vi "LV_client_port_DAQ - sh 4 outputs.vi"() -> ()   [LabVIEW 2014]
uses:
  <vilib>/DAQmx/create/channels.llb/DAQmx Create Channel (AO-Voltage-Basic).vi
  <vilib>/DAQmx/configure/timing.llb/DAQmx Timing (Sample Clock).vi
  <vilib>/DAQmx/configure/trigger.llb/DAQmx Start Trigger (None).vi
  <vilib>/DAQmx/write.llb/DAQmx Write (Analog 1D DBL NChan 1Samp).vi
panel:
  in  "mode":T1(ring)=enum."Immediate"
  in  "Yaw Constant":dbl=1800.0
  in  "Forward Constnt":dbl=1800.0
  out "Forward":dbl(graph)
  out "Yaw":dbl(graph)
  in  "Vthresh":dbl=0.1
  in  "forward\noffset":dbl=-0.019 format="%_4f"
  in  "Yaw\nOffset":dbl=-0.019 format="%_4f"
  out "Forward 2":dbl(graph)
  out "Yaw 2":dbl(graph)
  in  "Stop":bool
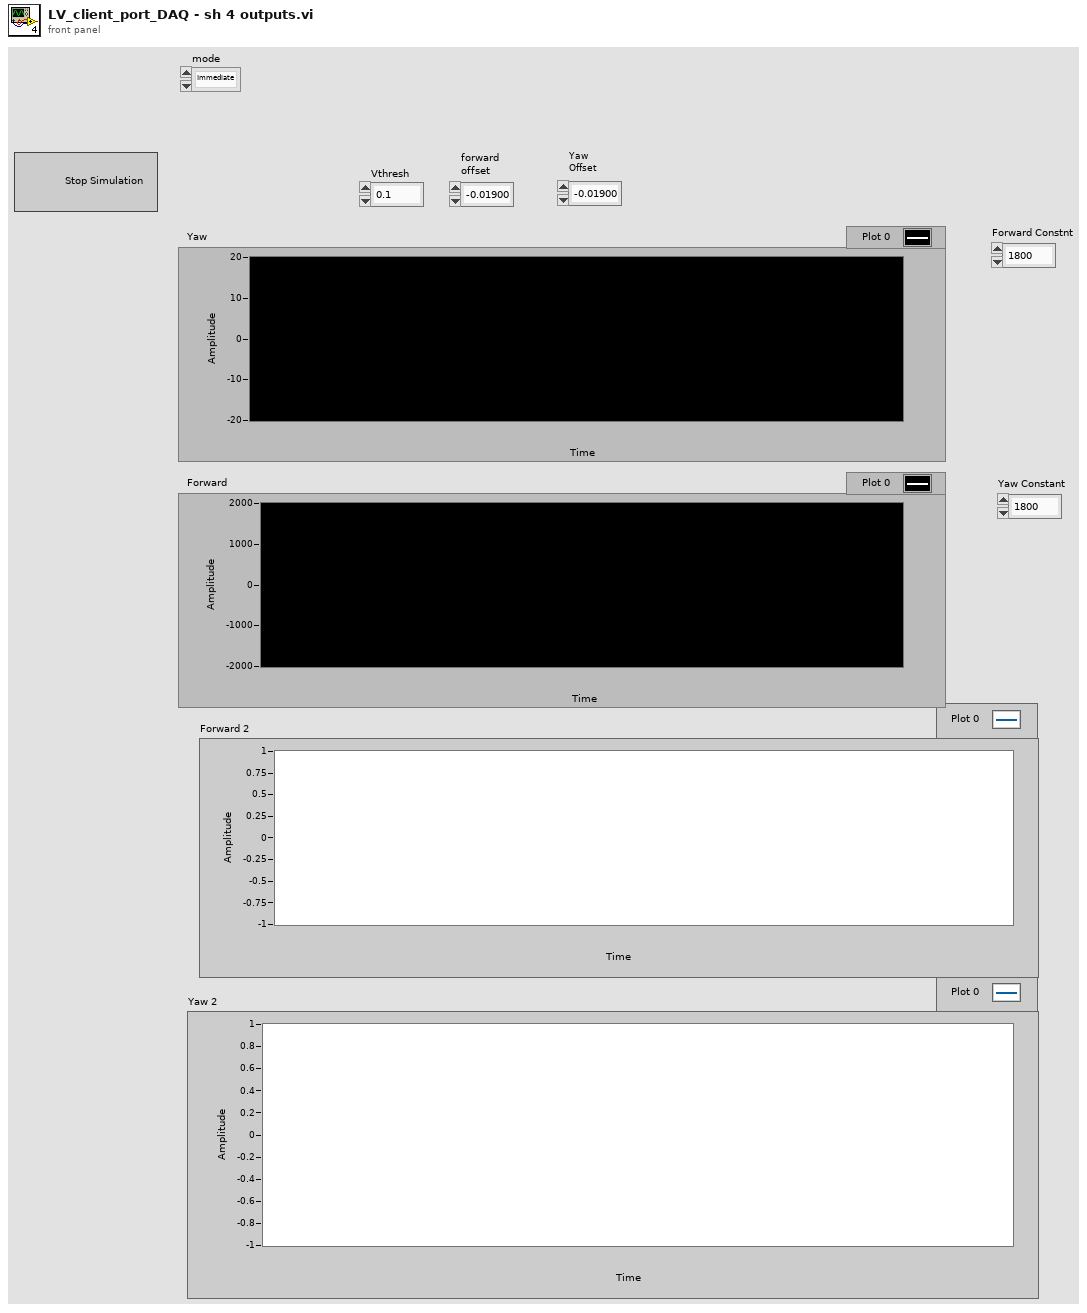
[diagram p1: front panel]
types:
  T1 = enum16{"Standard", "Buffered", "CRLF", "Immediate"}
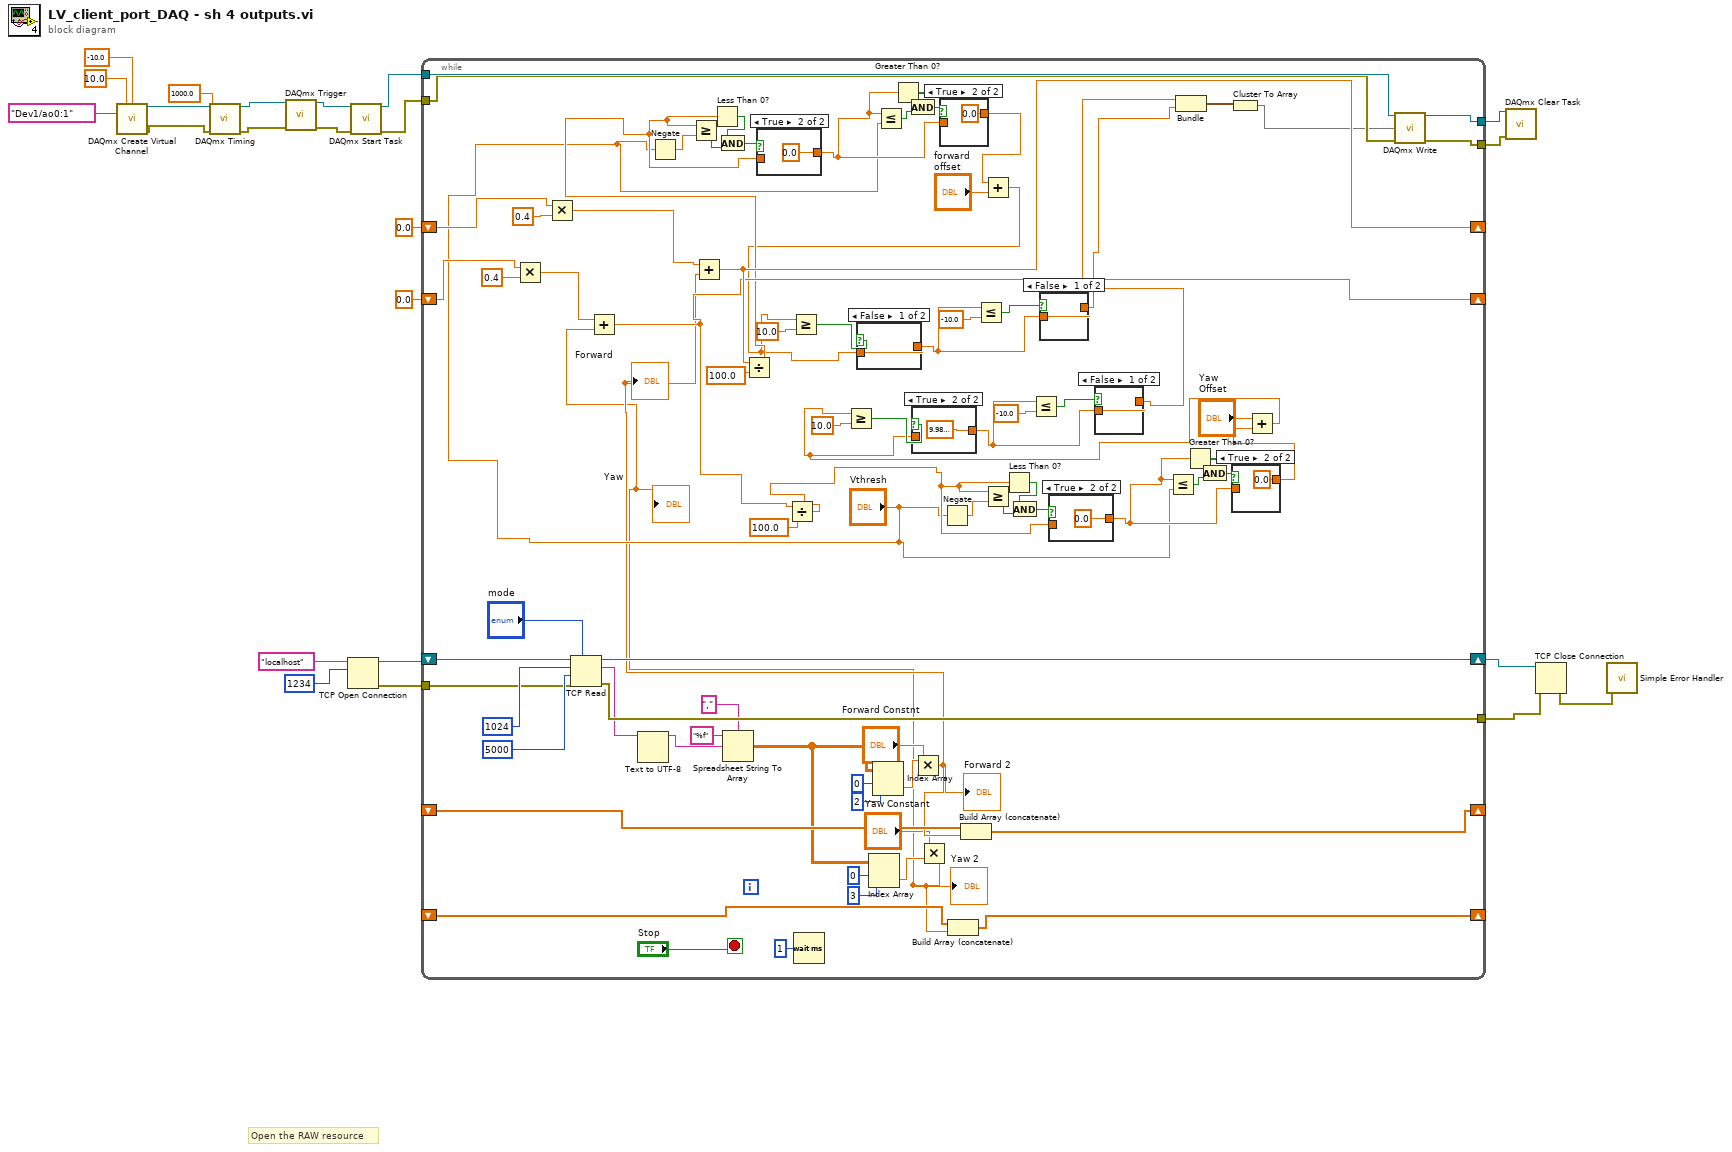
[diagram p0: block diagram]
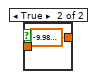
[diagram p6: hidden frame]
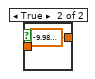
[diagram p8: hidden frame]
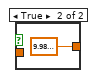
[diagram p9: hidden frame]
diagram:
  # "Open the RAW resource"
  n1 = call-poly <vilib>:"DAQmx Create Virtual Channel.vi"("maximum value"=10.0, "minimum value"=-10.0, "physical channels"=tag "Dev1/ao0:1") -> ("task out"=w21:refnum<k21>, "error out"=w20:errorcluster)  [unwired: 11 in]
  n2 = call-poly <vilib>:"DAQmx Timing.vi"("task/channels in"=w21, "rate"=1000.0, "error in"=w20) -> ("task out"=w19:refnum<k21>, "error out"=w18:errorcluster)  [unwired: 11 in]
  n3 = call-poly <vilib>:"DAQmx Trigger.vi"("task/channels in"=w19, "error in"=w18) -> ("task out"=w17:refnum<k21>, "error out"=w16:errorcluster)  [unwired: 12 in]
  n4 = TCP Open Connection(address="localhost", remote port or service name=u16 1234) -> (connection ID=w5:refnum<k5>, error out=w4:errorcluster)  [unwired: 3 in]
  n5 = call <vilib>:"DAQmx Start Task.vi"("task/channels in"=w17, "error in"=w16) -> ("task out"=w11:refnum<k21>, "error out"=w10:errorcluster)  [unwired: 12 in]
  n6 = while {
    shift-right: [w90] -> _
    shift-left: 0.0 -> [w91]
    shift-right: [w86] -> _
    shift-left: 0.0 -> [w87]
    tunnel: w11 -> [w59]
    tunnel: w10 -> [w58]
    tunnel: [w61] -> w9
    tunnel: [w60] -> w8
    tunnel: [w41] -> w3
    shift-right: [w40] -> w1
    shift-left: w5 -> [w46]
    shift-right: [w50] -> _
    shift-left: _ -> [w51]
    shift-right: [w48] -> _
    shift-left: _ -> [w49]
    tunnel: w4 -> [w43]
    stop <- "Stop" stop-if-true
    n7 = Multiply(x=w87, y=0.4) -> (x*y=w89:dbl)
    n8 = Multiply(x=w91, y=0.4) -> (x*y=w93:dbl)
    n9 = TCP Read(connection ID=w46, bytes to read=1024, error in (no error)=w43, 7:"mode", 9:5000 ("timeout ms (25000)")) -> (connection ID out=w40:refnum<k5>, data out=w39:string, error out=w41:errorcluster)
    n10 = Text to UTF-8(11:w39) -> (3:w38:string)  [unwired: 2 in, 1 out]
    n11 = Negate(x="Vthresh") -> (-x=w77:dbl)
    n12 = Spreadsheet String To Array(delimiter (Tab)=",", format string="%f", spreadsheet string=w38) -> (array=w33:dbl[][])  [unwired: 1 in]
    n13 = Wait (ms)(milliseconds to wait=u32 1) -> ()  [unwired: 1 out]
    n14 = Index Array(array=w33, index (row)=0, index (col)=3 ("disabled index (col)")) -> (element=w27:dbl)
    n15 = Index Array(array=w33, index (row)=0, index (col)=2 ("disabled index (col)")) -> (element=w30:dbl)
    n16 = Multiply(x=w30, y="Forward Constnt") -> (x*y=w28:dbl)
    "Forward" <- w28
    "Forward 2" <- w28
    n17 = Add(x=w93, y=w28) -> (x+y=w90:dbl)
    n18 = Divide(x=w90, y=sgl 100.0) -> (x/y=w68:dbl)
    n19 = Greater Or Equal?(x=w68, y=w77) -> (x >= y?=w74:bool)
    n20 = Less Than 0?(x=w68) -> (x < 0?=w75:bool)
    n21 = And(x=w75, y=w74) -> (x .and. y?=w76:bool)
    n22 = case shown="True" w76 {
      tunnel: [w107 sgl 0.0 ("y")] -> w73
      tunnel: w68 -> [w107 _]
      frame False {
      }
      frame True {
      }
    }
    n23 = Less Or Equal?(x=w73, y="Vthresh") -> (x <= y?=w71:bool)
    n24 = Greater Than 0?(x=w73) -> (x > 0?=w72:bool)
    n25 = And(x=w72, y=w71) -> (x .and. y?=w70:bool)
    n26 = Multiply(x="Yaw Constant", y=w27) -> (x*y=w25:dbl)
    "Yaw" <- w25
    "Yaw 2" <- w25
    n27 = Add(x=w89, y=w25) -> (x+y=w86:dbl)
    n28 = Divide(x=w86, y=sgl 100.0) -> (x/y=w69:dbl)
    n29 = case shown="True" w70 {
      tunnel: [w105 sgl 0.0 ("y")] -> w67
      tunnel: w73 -> [w105 _]
      frame False {
      }
      frame True {
      }
    }
    n30 = Negate(x="Vthresh") -> (-x=w53:dbl)
    n31 = Build Array (concatenate)(w49, w25) -> (w48:dbl[])
    n32 = Build Array (concatenate)(w51, w28) -> (w50:dbl[])
    n33 = Add(x=w67, y="forward\noffset") -> (x+y=w65:dbl)
    n34 = Greater Or Equal?(x=w65, y=sgl 10.0) -> (x >= y?=w103:bool)
    n35 = case shown="False" w103 {
      tunnel: [w119 sgl 9.99 ("y")] -> w99
      tunnel: w65 -> [w119 _]
      frame False {
      }
      frame True {
      }
    }
    n36 = Less Or Equal?(x=w99, y=sgl -10.0) -> (x <= y?=w100:bool)
    n37 = Greater Or Equal?(x=w69, y=w53) -> (x >= y?=w82:bool)
    n38 = Less Than 0?(x=w69) -> (x < 0?=w83:bool)
    n39 = And(x=w83, y=w82) -> (x .and. y?=w84:bool)
    n40 = case shown="False" w100 {
      tunnel: [w117 sgl -9.99 ("y")] -> w54
      tunnel: w99 -> [w117 _]
      frame False {
      }
      frame True {
      }
    }
    n41 = case shown="True" w84 {
      tunnel: [w111 sgl 0.0 ("y")] -> w81
      tunnel: w69 -> [w111 _]
      frame False {
      }
      frame True {
      }
    }
    n42 = Less Or Equal?(x=w81, y="Vthresh") -> (x <= y?=w79:bool)
    n43 = Greater Than 0?(x=w81) -> (x > 0?=w80:bool)
    n44 = And(x=w80, y=w79) -> (x .and. y?=w78:bool)
    n45 = case shown="True" w78 {
      tunnel: [w109 sgl 0.0 ("y")] -> w66
      tunnel: w81 -> [w109 _]
      frame False {
      }
      frame True {
      }
    }
    n46 = Add(x="Yaw\nOffset", y=w66) -> (x+y=w63:dbl)
    n47 = Greater Or Equal?(x=w63, y=sgl 10.0) -> (x >= y?=w85:bool)
    n48 = case shown="True" w85 {
      tunnel: [w115 sgl 9.99 ("y")] -> w95
      tunnel: w63 -> [w115 _]
      frame False {
      }
      frame True {
      }
    }
    n49 = Less Or Equal?(x=w95, y=sgl -10.0) -> (x <= y?=w96:bool)
    n50 = case shown="False" w96 {
      tunnel: [w113 sgl -9.99 ("y")] -> w55
      tunnel: w95 -> [w113 _]
      frame False {
      }
      frame True {
      }
    }
    n51 = Bundle("y"=w55, "y"=w54) -> (w57:cluster{"y":dbl, "y":dbl})  [unwired: 1 in]
    n52 = Cluster To Array(cluster=w57) -> (array=w56:dbl[])
    n53 = call-poly <vilib>:"DAQmx Write.vi"("task/channels in"=w59, "data"=w56, "error in"=w58) -> ("task out"=w61:refnum<k21>, "error out"=w60:errorcluster)  [unwired: 10 in, 1 out]
  }
  n54 = call <vilib>:"DAQmx Clear Task.vi"("task in"=w9, "error in"=w8) -> ()  [unwired: 13 in, 1 out]
  n55 = TCP Close Connection(connection ID=w1, error in (no error)=w3) -> (error out=w2:errorcluster)  [unwired: 1 in, 1 out]
  n56 = call <vilib>:"Simple Error Handler.vi"("error in (no error)"=w2) -> ()  [unwired: 1 in, 8 out]
